vi "ITC503 Get Values.vi"(3 "ITC Setup":T2={"Description"="", "IO Info"={"Address"={"Com Port"=1, "ISOBUS Address"=1, "GPIB Address"=24, "Communication"=enum."ISOBUS"}, "Version"=enum."ITC503", "Ch 1 dec places"=1, "Ch 2 dec places"=1, "Ch 3 dec places"=1, "Ch1 Name"="", "Ch2 Name"="", "Ch3 Name"=""}}) -> (0 "Control Channel":i16, 1 "ITC503 Current Values":T1 {"ITC503 Gradient" format="%.2f"; "ITC503 Setpoint" min=-273.0 max=300000.0 step=0.0001 format="%.1f"; "ITC503 I" format="%_1f"; "ITC503 P" format="%_1f"; "ITC503 Temperature" min=0.0 max=1645.0 step=1e-05 format="%.2f"; "ITC503 Heater" min=0.0 max=100.0 step=0.01 scale=0.0..100.0})   [LabVIEW 2010]
uses:
  drivers/Oxford ITC/ITCAPPS.LLB/ITCSetup.ctl
  drivers/Oxford ITC/ITCSUBS.LLB/ITCIO.ctl
  drivers/Oxford ITC/BUSGEN.LLB/OxfordAddress.ctl
  drivers/Oxford ITC/ITCSUBS.LLB/ITCVersion.ctl
  TypeDefs/ITC503 Current Values.ctl
panel:
  out "Gas Is Auto":bool
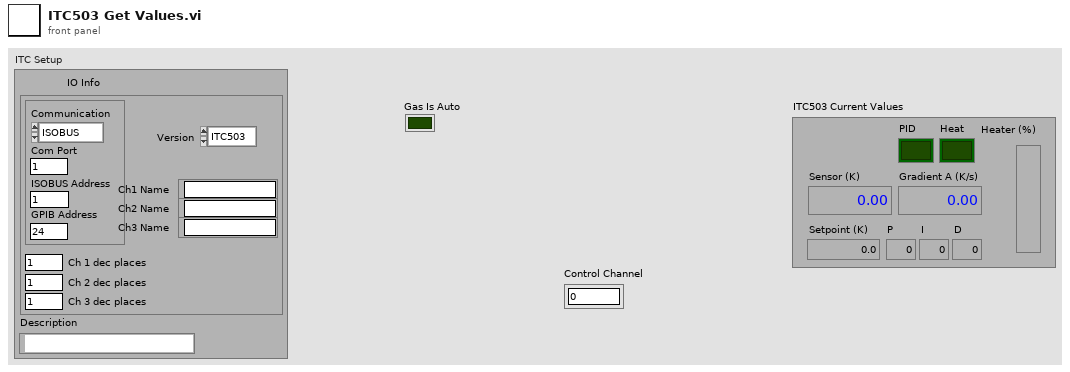
[diagram p1: front panel]
types:
  T1 = typedef "ITC503 Current Values.ctl" = cluster{"ITC503 Heater":dbl, "ITC503 Temperature":dbl, "ITC503 P":dbl, "ITC503 I":dbl, "ITC503 D":dbl, "ITC503 Setpoint":dbl, "ITC503 Gradient":dbl, "ITC503 Heater Auto":bool, "ITC503 PID Auto":bool}
  T2 = typedef "ITCSetup.ctl" = cluster{"Description":string, "IO Info":T3}
  T3 = typedef "ITCIO.ctl" = cluster{"Address":T4, "Version":T5, "Ch 1 dec places":i16, "Ch 2 dec places":i16, "Ch 3 dec places":i16, "Ch1 Name":string, "Ch2 Name":string, "Ch3 Name":string}
  T4 = typedef "OxfordAddress.ctl" = cluster{"Com Port":i32, "ISOBUS Address":i32, "GPIB Address":i16, "Communication":enum16{"RS232", "ISOBUS", "GPIB", "Gateway"}}
  T5 = typedef "ITCVersion.ctl" = enum16{"ITC502", "ITC503", "ITC601"}
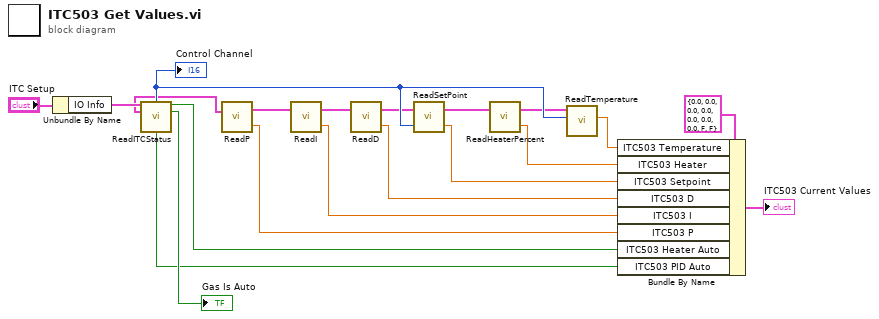
[diagram p0: block diagram]
diagram:
  n1 = Unbundle By Name("ITC Setup") -> ("IO Info"=w18:T3)
  n2 = call "ReadITCStatus.vi"("ITC IO Info"=w18) -> ("Control Channel"=w20:i16, "Auto heat"=w9:bool, "ITC IO Info"=w14:T3, "Auto Needle Valve"=→"Gas Is Auto":bool, "Auto PID"=w8:bool)  [unwired: 4 in, 6 out]
  "Control Channel" <- w20
  n3 = call "ReadP.vi"("IO Info"=w14) -> ("Actual P (% of span)"=w7:dbl, "ITC IO Info"=w16:T3)  [unwired: 1 in]
  n4 = call "ReadI.vi"("IO Info"=w16) -> ("Actual I"=w6:dbl, "ITC IO Info"=w15:T3)  [unwired: 1 in]
  n5 = call "ReadD.vi"("IO Info"=w15) -> ("Actual D"=w5:dbl, "ITC IO Info"=w13:T3)  [unwired: 1 in]
  n6 = call "ReadSetPoint.vi"("Control Ch"=w20, "IO Info"=w13) -> ("Set point"=w2:dbl, "ITC IO Info"=w12:T3)
  n7 = call "ReadHeaterPercent.vi"("ITC IO Info"=w12) -> ("Actual heater  %"=w3:dbl, "ITC IO Info"=w11:T3)  [unwired: 1 in]
  n8 = call "ReadTemperature.vi"("Channel"=w20, "IO Info"=w11) -> ("Temperature"=w4:dbl)  [unwired: 3 in, 2 out]
  n9 = Bundle By Name(cluster=T1 {"ITC503 Heater"=0.0, "ITC503 Temperature"=0.0, "ITC503 P"=0.0, "ITC503 I"=0.0, "ITC503 D"=0.0, "ITC503 Setpoint"=0.0, "ITC503 Gradient"=0.0, "ITC503 Heater Auto"=FALSE, "ITC503 PID Auto"=FALSE} ("ITC503 Current Values"), "ITC503 Temperature"=w4, "ITC503 Heater"=w3, "ITC503 Setpoint"=w2, "ITC503 D"=w5, "ITC503 I"=w6, "ITC503 P"=w7, "ITC503 Heater Auto"=w9, "ITC503 PID Auto"=w8) -> (→"ITC503 Current Values":T1)
